vi "UpdateSettings.verticaloffset.vi"(8 "error in (no error)":errorcluster, 10 "ChannelName":string, 11 "TektronixDPO in":refnum<class "TektronixDPO.lvclass">) -> (0 "error out":errorcluster, 3 "TektronixDPO out":refnum<class "TektronixDPO.lvclass">)   [LabVIEW 2013, in "TektronixDPO.lvclass"]
uses:
  TektronixDPO.lvclass
  settings_TypDef.ctl
  shared/numericVariable_TypeDef.ctl
  shared/OnOffTypeDef.ctl
  PXIdigitizer/subVis/analysisTypDEf.ctl
  PXIdigitizer/subVis/additionalAnalysisCluster_TypDef.ctl
  PXIdigitizer/subVis/LinkedChannelsCluster_TypDef.ctl
  PXIdigitizer/subVis/channels_TypDef.ctl
  PXIdigitizer/subVis/methodCluster_TypDEf.ctl
  ScopeAnalysis/SubVis/method_TypDef.ctl
  TypeDefs/TriggerCluster.ctl
  shared/Typdefs/Choice73.ctl
  shared/Typdefs/Choice74.ctl
  shared/Typdefs/Choice75.ctl
  shared/Typdefs/Choice76.ctl
  TypeDefs/Horizontal.ctl
  shared/Typdefs/Choice77.ctl
  shared/Typdefs/Choice78.ctl
  shared/Typdefs/Choice79.ctl
  shared/Typdefs/Choice11.ctl
  TektronixDPO.lvclass/TektronixDPO.ctl
  SupportClasses/TektronixDPOPhysicalDevice/TektronixDPO_PhysicalDevice.lvclass
  BaseDriver/BaseDriver.lvclass
panel:
  in  "Settings":T1={"resourcename"="", "timeout"={"Value"=0.0, "Min"=0.0, "Max"=0.0, "StepSize"=0.0, "Tolerance"=0.0, "ValueActual"=0.0}, "LocalSavingPath"=path "", "Save"=enum."off", "Names"={"Channel0"="", "Channel1"="", "Channel2"="", "Channel3"="", "Channel4"=""}, "Calculations"={"Additional"={"Analysis1"=0.0, "Analysis2"=0.0, "Analysis3"=0.0, "Analysis4"=0.0, "Analysis5"=0.0, "Analysis6"=0.0, "Analysis7"=0.0, "Analysis8"=0.0, "Analysis9"=0.0, "Analysis10"=0.0}, "Linked"={"Analysis1"=enum."Channel0", "Analysis2"=enum."Channel0", "Analysis3"=enum."Channel0", "Analysis4"=enum."Channel0", "Analysis5"=enum."Channel0", "Analysis6"=enum."Channel0", "Analysis7"=enum."Channel0", "Analysis8"=enum."Channel0", "Analysis9"=enum."Channel0", "Analysis10"=enum."Channel0"}, "Method"={"Analysis1"=enum."max", "Analysis2"=enum."max", "Analysis3"=enum."max", "Analysis4"=enum."max", "Analysis5"=enum."max", "Analysis6"=enum."max", "Analysis7"=enum."max", "Analysis8"=enum."max", "Analysis9"=enum."max", "Analysis10"=enum."max"}}, "NumChannels"={"Value"=0.0, "Min"=0.0, "Max"=0.0, "StepSize"=0.0, "Tolerance"=0.0, "ValueActual"=0.0}, "NumMeasurements"={"Value"=0.0, "Min"=0.0, "Max"=0.0, "StepSize"=0.0, "Tolerance"=0.0, "ValueActual"=0.0}, "NumPoints"={"Value"=0.0, "Min"=0.0, "Max"=0.0, "StepSize"=0.0, "Tolerance"=0.0, "ValueActual"=0.0}, "waveformattributes"="waveformattributes>>force", "Measurements"={"Channel0"={"Value"=0.0, "Min"=0.0, "Max"=0.0, "StepSize"=0.0, "Tolerance"=0.0, "ValueActual"=0.0}, "Channel1"={"Value"=0.0, "Min"=0.0, "Max"=0.0, "StepSize"=0.0, "Tolerance"=0.0, "ValueActual"=0.0}, "Channel2"={"Value"=0.0, "Min"=0.0, "Max"=0.0, "StepSize"=0.0, "Tolerance"=0.0, "ValueActual"=0.0}, "Channel3"={"Value"=0.0, "Min"=0.0, "Max"=0.0, "StepSize"=0.0, "Tolerance"=0.0, "ValueActual"=0.0}}, "EnableMeasurements"=enum."off", "Trigger"={"Mode"=enum."Immediate", "Source"=enum."Channel 1", "Coupling"=enum."DC", "Slope"=enum."Rising", "Low Level"=0.0}, "EnableReadWaveformInfo"=enum."off", "probeattenuation"={"Channel0"={"Value"=0.0, "Min"=0.0, "Max"=0.0, "StepSize"=0.0, "Tolerance"=0.0, "ValueActual"=0.0}, "Channel1"={"Value"=0.0, "Min"=0.0, "Max"=0.0, "StepSize"=0.0, "Tolerance"=0.0, "ValueActual"=0.0}, "Channel2"={"Value"=0.0, "Min"=0.0, "Max"=0.0, "StepSize"=0.0, "Tolerance"=0.0, "ValueActual"=0.0}, "Channel3"={"Value"=0.0, "Min"=0.0, "Max"=0.0, "StepSize"=0.0, "Tolerance"=0.0, "ValueActual"=0.0}}, "offset"={"Channel0"={"Value"=0.0, "Min"=0.0, "Max"=0.0, "StepSize"=0.0, "Tolerance"=0.0, "ValueActual"=0.0}, "Channel1"={"Value"=0.0, "Min"=0.0, "Max"=0.0, "StepSize"=0.0, "Tolerance"=0.0, "ValueActual"=0.0}, "Channel2"={"Value"=0.0, "Min"=0.0, "Max"=0.0, "StepSize"=0.0, "Tolerance"=0.0, "ValueActual"=0.0}, "Channel3"={"Value"=0.0, "Min"=0.0, "Max"=0.0, "StepSize"=0.0, "Tolerance"=0.0, "ValueActual"=0.0}}, "Horizontal"={"time_window"=10000000.0, "resolution"=enum."10E+6"}, "verticalrange"={"Channel0"={"Value"=0.0, "Min"=0.0, "Max"=0.0, "StepSize"=0.0, "Tolerance"=0.0, "ValueActual"=0.0}, "Channel1"={"Value"=0.0, "Min"=0.0, "Max"=0.0, "StepSize"=0.0, "Tolerance"=0.0, "ValueActual"=0.0}, "Channel2"={"Value"=0.0, "Min"=0.0, "Max"=0.0, "StepSize"=0.0, "Tolerance"=0.0, "ValueActual"=0.0}, "Channel3"={"Value"=0.0, "Min"=0.0, "Max"=0.0, "StepSize"=0.0, "Tolerance"=0.0, "ValueActual"=0.0}}, "Impedance"={"Channel0"=enum."1M", "Channel1"=enum."1M", "Channel2"=enum."1M", "Channel3"=enum."1M"}, "channelenabled"={"Channel0"=enum."off", "Channel1"=enum."off", "Channel2"=enum."off", "Channel3"=enum."off"}, "bandwidth"={"Channel0"=enum."FULL", "Channel1"=enum."FULL", "Channel2"=enum."FULL", "Channel3"=enum."FULL"}, "coupling"={"Channel0"=enum."DC", "Channel1"=enum."DC", "Channel2"=enum."DC", "Channel3"=enum."DC"}} {"Horizontal"."time_window" step=1000000.0 format="%.2p"}
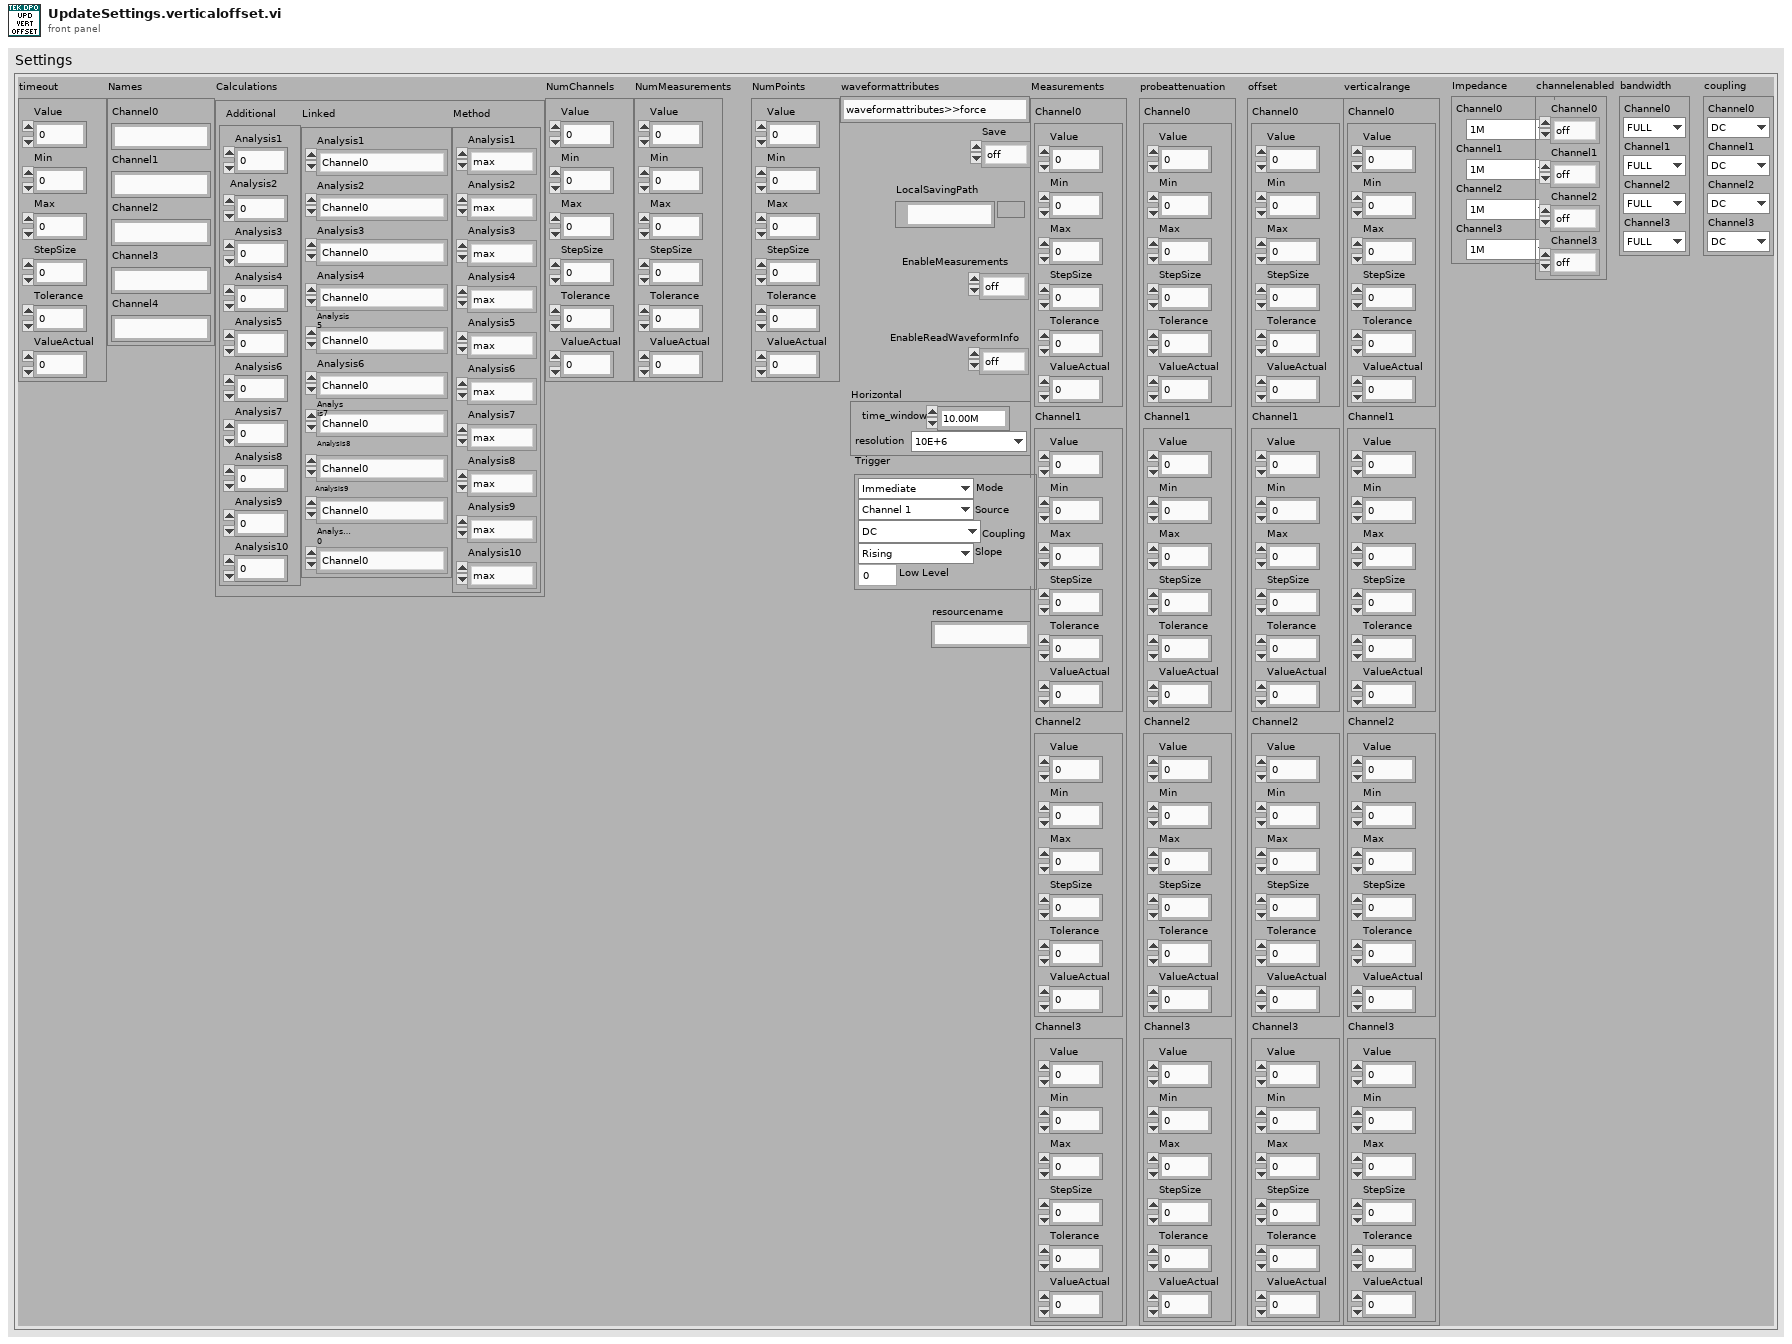
[diagram p1: front panel]
types:
  T1 = typedef "settings_TypDef.ctl" = cluster{"resourcename":string, "timeout":T2, "LocalSavingPath":path, "Save":T3, "Names":cluster{"Channel0":string, "Channel1":string, "Channel2":string, "Channel3":string, "Channel4":string}, "Calculations":T4, "NumChannels":T2, "NumMeasurements":T2, "NumPoints":T2, "waveformattributes":string, "Measurements":cluster{"Channel0":T2, "Channel1":T2, "Channel2":T2, "Channel3":T2}, "EnableMeasurements":T3, "Trigger":T10, "EnableReadWaveformInfo":T3, "probeattenuation":cluster{"Channel0":T2, "Channel1":T2, "Channel2":T2, "Channel3":T2}, "offset":cluster{"Channel0":T2, "Channel1":T2, "Channel2":T2, "Channel3":T2}, "Horizontal":T15, "verticalrange":cluster{"Channel0":T2, "Channel1":T2, "Channel2":T2, "Channel3":T2}, "Impedance":cluster{"Channel0":T17, "Channel1":T17, "Channel2":T17, "Channel3":T17}, "channelenabled":cluster{"Channel0":T3, "Channel1":T3, "Channel2":T3, "Channel3":T3}, "bandwidth":cluster{"Channel0":T18, "Channel1":T18, "Channel2":T18, "Channel3":T18}, "coupling":cluster{"Channel0":T19, "Channel1":T19, "Channel2":T19, "Channel3":T19}}
  T2 = typedef "BaseDriver.lvclass/numericVariable_TypeDef.ctl" = cluster{"Value":dbl, "Min":dbl, "Max":dbl, "StepSize":dbl, "Tolerance":dbl, "ValueActual":dbl}
  T3 = typedef "OnOffTypeDef.ctl" = enum16{"off", "on"}
  T4 = typedef "analysisTypDEf.ctl" = cluster{"Additional":T5, "Linked":T6, "Method":T8}
  T5 = typedef "additionalAnalysisCluster_TypDef.ctl" = cluster{"Analysis1":dbl, "Analysis2":dbl, "Analysis3":dbl, "Analysis4":dbl, "Analysis5":dbl, "Analysis6":dbl, "Analysis7":dbl, "Analysis8":dbl, "Analysis9":dbl, "Analysis10":dbl}
  T6 = typedef "LinkedChannelsCluster_TypDef.ctl" = cluster{"Analysis1":T7, "Analysis2":T7, "Analysis3":T7, "Analysis4":T7, "Analysis5":T7, "Analysis6":T7, "Analysis7":T7, "Analysis8":T7, "Analysis9":T7, "Analysis10":T7}
  T7 = typedef "channels_TypDef.ctl" = enum16{"Channel0", "Channel1", "Channel2", "Channel3", "Channel4", "Channel5", "Channel6", "Channel7", "n/a"}
  T8 = typedef "methodCluster_TypDEf.ctl" = cluster{"Analysis1":T9, "Analysis2":T9, "Analysis3":T9, "Analysis4":T9, "Analysis5":T9, "Analysis6":T9, "Analysis7":T9, "Analysis8":T9, "Analysis9":T9, "Analysis10":T9}
  T9 = typedef "method_TypDef.ctl" = enum16{"n/a", "max", "min", "energy", "trigger", "maxtime", "mintime"}
  T10 = typedef "TriggerCluster.ctl" = cluster{"Mode":T11, "Source":T12, "Coupling":T13, "Slope":T14, "Low Level":dbl}
  T11 = typedef "Choice73.ctl" = enum16{"Immediate", "Analog Edge"}
  T12 = typedef "Choice74.ctl" = enum16{"Channel 1", "Channel 2", "Channel 3", "Channel 4", "AC Line", "Aux", "Digital Channel 0", "Digital Channel 1", "Digital Channel 2", "Digital Channel 3", "Digital Channel 4", "Digital Channel 5", "Digital Channel 6", "Digital Channel 7", "Digital Channel 8", "Digital Channel 9", "Digital Channel 10", "Digital Channel 11", "Digital Channel 12", "Digital Channel 13", "Digital Channel 14", "Digital Channel 15", "RF"}
  T13 = typedef "Choice75.ctl" = enum16{"DC", "HF Reject", "LF Reject", "Noise Reject", "AC"}
  T14 = typedef "Choice76.ctl" = enum16{"Rising", "Falling"}
  T15 = typedef "Horizontal.ctl" = cluster{"time_window":dbl, "resolution":T16}
  T16 = typedef "Choice77.ctl" = enum16{"1E+3", "10E+3", "100E+3", "1E+6", "5E+6", "10E+6"}
  T17 = typedef "Choice78.ctl" = enum16{"1M", "75", "50"}
  T18 = typedef "Choice79.ctl" = enum16{"FULL", "250 MHz", "150 MHz", "20 MHz"}
  T19 = typedef "Choice11.ctl" = enum16{"AC", "DC", "Ground"}
  T20 = typedef "Choice78.ctl" = u16
  T21 = cluster{"Channel":T20, "offset":dbl, "verticalrange":dbl, "Impedance":u16, "Probe Attenuation":dbl, "Vertical Coupling":u16, "Bandwidth":u16, "Enabled":bool}
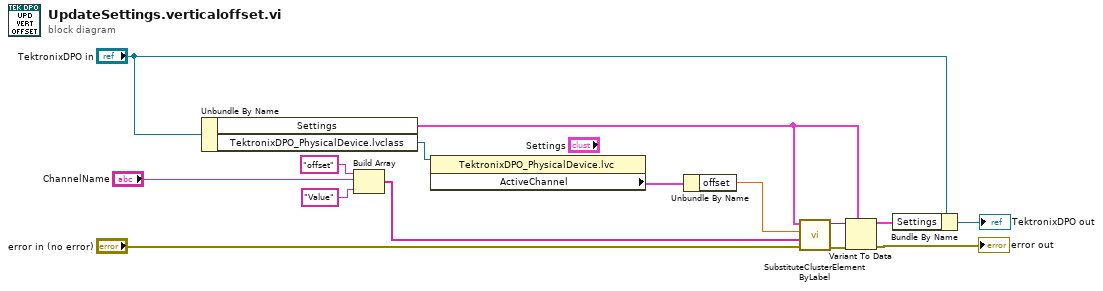
[diagram p0: block diagram]
diagram:
  n1 = Unbundle By Name("TektronixDPO in") -> ("Settings"=w1:T1, "TektronixDPO_PhysicalDevice.lvclass"=w8:refnum<class "TektronixDPO_PhysicalDevice.lvclass">)
  n2 = Build Array("offset" ("Element Name"), "ChannelName", "Value" ("Element Name")) -> (w7:string[])
  n3 = property class="TektronixDPO_PhysicalDevice.lvc"(reference=w8) -> ("ActiveChannel"=w9:T21)  [unwired: 1 in, 2 out]
  n4 = Unbundle By Name(w9) -> ("offset"=w2:dbl)
  n5 = call "SubstituteClusterElementByLabel.vi"("error in (no error)"="error in (no error)", "ElementHierarchy"=w7, "NewElementValue"=w2, "ClusterIn"=w1) -> ("ErrorOut"=w10:errorcluster, "UpdatedClusterOut"=w11:variant)  [unwired: 5 in, 1 out]
  n6 = Variant To Data(error in=w10, type=w1, Variant=w11) -> (data=w12:T1, error out=→"error out":errorcluster)
  n7 = Bundle By Name(cluster="TektronixDPO in", "Settings"=w12) -> (→"TektronixDPO out":refnum<class "TektronixDPO.lvclass">)
